vi "SteuerungWaermepumpe_DhruvTest.vi"() -> ()   [LabVIEW 2015]
uses:
  <vilib>/DAQmx/read.llb/DAQmx Read (Analog 1D Wfm NChan NSamp).vi
  <vilib>/DAQmx/write.llb/DAQmx Write (Analog 1D Wfm NChan 1Samp).vi
  <vilib>/MakerHub/LINX/Public/Peripherals/Digital/Digital Write N Chans.vi
  <vilib>/MakerHub/LINX/Private/Local IO/LinxDigitalWrite.vi
  <vilib>/MakerHub/LINX/Public/Utilities/Check Channel.vi
  <vilib>/MakerHub/LINX/Private/Utilties/Generate Error.vi
  <vilib>/DAQmx/miscellaneous.llb/DAQmx Fill In Error Info.vi
  <vilib>/Utility/file.llb/Read Delimited Spreadsheet (DBL).vi
  <vilib>/MakerHub/LINX/LMH-LINX.lvlib
panel:
  in  "stop":bool
  out "x = y?":bool
  out "concatenated string":string
  out "Number of Thermocouples":dbl
  out "Keithley Temperature Graph":waveform(dbl)[](graph)
  out "error out":errorcluster
  out "Array 2":dbl[](array[numeric])
  out "Abscheider":cluster{dbl, dbl, dbl}(slide) scale=0.0..1.3
  in  "Rampe":bool=TRUE
  in  "Rampe rpm/s":dbl=1.0 min=1.0 max=100.0 step=1.0
  out "Rampe IW":dbl
  in  "reinitialize HD":bool
  in  "reinitialize Pumpe":bool
  out "ist an!":string
  in  "zusätzlicher Druck":dbl
  in  "PI05 SW":dbl format="%.2f"
  out "p_liq_mittel":dbl
  out "p_liq":dbl
  out "Schleifendauer":dbl format="%.5f"
  out "Mittelwert 2":dbl
  in  "Mittelwert HD":bool
  in  "Mittelwert Pumpe":bool
  out "Mittelwert":dbl
  in  "Xi / p_liq berechnung an":bool
  out "xi_r":dbl
  in  "Regler Senke":bool
  in  "reinitialize Senke":bool
  in  "TI35 SW":dbl=43.0 format="%.2f"
  in  "Drehzahl Bestätigung":bool
  in  "Drehzahl SW":dbl=1000.0 min=500.0 max=3000.0 step=1.0 format="%#_4g"
  out "Check":dbl format="%#_13g"
  in  "Regler Hochdruck":bool
  in  "PID Regelung Pumpe":bool
  in  "SW TI39":dbl
  out "Array":bool[](array[boolean])
  in  "LEDs 2":bool[](array[boolean])
  in  "Regelung HK":bool
  in  "RV 30 zu":bool
  in  "RV 30 auf":bool
  out "FI_Oel":dbl
  in  "RV 33":dbl(slide) scale=-1.0..1.0
  in  "tag":string
  out "Pumpenwerte":dbl[](array[numeric]) format="%.2f"
  out "Speichert!":bool
  out "Historie":string
  in  "Kommentar":string
  out "refnum out":refnum<file>
  in  "Identität!":string(combo)
  in  "Zeit X in Minuten":dbl(slide)=5.0 min=0.0 max=15.0 scale=5.0..15.0
  out "TI 21a Warnungen":dbl
  out "Leistung":dynamicdata(graph)
  out "TI 37":dbl
  in  "Programm stoppen!":bool
  out "%":sgl(slide) scale=0.0..100.0
  out "kalt":bool
  out "warm":bool
  out "?":T1(array[cluster]) {"?" format="%#.4g"; "Konzentration_reich" format="%#.4g"}
  in  "Mit EES vergleichen":bool
  in  "FI13 SW in l/min":dbl=3.0 min=3.0 max=12.0 step=0.10000000149011612
  out "COP_Oel":dbl
  out "Q-Oel kW":dbl format="%_4g"
  in  "Dateiname!":string
  in  "Comment":bool
  in  "Speichern":bool caption="Aktivieren"
  out "ZU     Ventilstellung 33     AUF":dbl(slide) scale=0.0..100.0 scale format="%.2f"
  in  "Regelventil 34":dbl(slide) min=0.0 max=100.0 step=0.009999999776482582 scale=0.0..100.0
  in  "Matlab":bool
  in  "?":T2(tab)
  out "?":dynamicdata(graph)
  out "?":waveform(dbl)(graph)
  out "?":dynamicdata(graph)
  out "PI 12":dbl format="%.2f"
  out "PI 11":dbl format="%.2f"
  out "Dichte":dbl format="%.5g"
  in  "Reset":bool
  out "Betriebszeit":cluster{"second":i32, "minute":i32, "hour":i32}
  out "Temperatur Ölprüfstand":dbl
  out "FI 13 kg/min":dbl
  in  "Messung\nFrequenzwandler":bool
  out "Magnetventil":bool
  out "Fl.Pumpe an":bool
  out "Temperatur Öl":bool
  out "COP":dbl format="%#_13g"
  out "Verdichteraktivität":cluster{"second":i32, "minute":i32, "hour":i32}
  out "Q-Entgaser kW":dbl format="%_4g"
  out "Warnungen":bool[](array[boolean])
  out "Status Komponenten":bool[](array[boolean])
  in  "Pumpen-Auto-Abschalt":bool=TRUE
  out "Q-Resorber kW":dbl format="%_4g"
  out "Stellung Expansionsventil":waveform(dbl)(graph)
  out "FI 35 l/min":dbl format="%#_13g"
  out "FI 38 l/min":dbl format="%#_13g"
  out "FI Oel l/min":dbl format="%#.3g"
  out "LI in l":dbl format="%#_4g"
  out "TI 39":dbl format="%#_3g"
  out "TI 38":dbl format="%#_3g"
  out "TI 36":dbl format="%#_3g"
  out "TI 35":dbl format="%#_3g"
  out "TI 33":dbl format="%#_3g"
  out "TI 32":dbl format="%#_3g"
  out "TI 34":dbl format="%#_3g"
  out "TI 21a":dbl format="%#_3g"
  out "TI 21":dbl format="%#_3g"
  out "TI 20":dbl format="%#_3g"
  out "TI 14a":dbl format="%#_3g"
  out "TI 14":dbl format="%#_3g"
  out "TI 13":dbl format="%#_3g"
  out "TI 12":dbl format="%#_3g"
  out "TI 11":dbl format="%#_3g"
  out "TI 10":dbl format="%#_3g"
  out "TI 09":dbl format="%#_3g"
  out "TI 08":dbl format="%#_3g"
  out "TI 07":dbl format="%#_3g"
  out "TI 06a":dbl format="%#_3g"
  out "TI 06":dbl format="%#_3g"
  out "TI 05":dbl format="%#_3g"
  out "TI 04":dbl format="%#_3g"
  out "TI 22":dbl format="%#_3g"
  out "TI 02":dbl format="%#_3g"
  out "TI 01":dbl format="%#_3g"
  out "Konzentration":dbl format="%#_5g"
  in  "Pumpensteuerung":dbl min=0.0 max=10.0 step=0.009999999776482582 format="%.2g"
  out "PI 08":dbl format="%.2f"
  out "PI 05":dbl format="%#.2f"
  out "PI 02":dbl format="%.2f"
  out "PI 04":dbl format="%.2f"
  out "PDI 8-9":dbl format="%.2f"
  out "PI 14":dbl format="%.2f"
  out "PI 01":dbl format="%.2f"
  out "ZU    Ventilstellung Exp.V     AUF":dbl(slide) scale=0.0..100.0 scale format="%#.1f"
  in  "Exp.V":dbl(slide)=3.0 min=0.0 max=100.0 step=1.0 scale=0.0..100.0 scale format="%#.0f"
  out "ZU    Ventilstellung 14      AUF":dbl(slide) caption="Auf    Ventilstellung 14      Zu" scale=0.0..100.0 scale format="%#.2f"
  in  "Regelventil 36":dbl(slide) min=0.0 max=100.0 step=0.009999999776482582 scale=0.0..100.0 scale format="%#.0f"
  out "ZU  Ventilstellung 35  AUF":dbl(slide) scale=0.0..100.0 scale format="%.2f"
  in  "Regelventil 35":dbl(slide)=100.0 min=0.0 max=100.0 step=0.009999999776482582 scale=0.0..100.0 scale format="%#.3g"
  out "ZU     Ventilstellung 39     AUF":dbl(slide) scale=0.0..100.0 scale format="%.2f"
  in  "Regelventil 39":dbl(slide)=100.0 min=0.0 max=100.0 step=0.009999999776482582 scale=0.0..100.0
  out "FI 13 l/min":dbl format="%.2f"
  out "FI 07 l/min":dbl format="%.2f"
  out "LI in m":dbl format="%.2f"
  out "PDI 5-6":dbl format="%.4f"
  out "PI 07":dbl format="%.2f"
  out "Druckverhältnis":dbl
  out "Drehzahl":dbl
  out "Drehmoment":dbl
  out "Frequenz":dbl
  out "Leistung":dbl
  out "Durchfluss":waveform(dbl)[](graph)
  in  "Tab Control Temperaturen":T3(tab)
  out "Temperatur Reich":waveform(dbl)[](graph)
  out "Temperatur Arm":waveform(dbl)[](graph)
  out "Temperatur Öl":waveform(dbl)[](graph)
  out "Temperatur Senke/Quelle":waveform(dbl)[](graph)
  out "Druck":waveform(dbl)[](graph)
  out "Druckzustand":bool caption="Zu viel Druck !!!"
  # "Öltemperatur"
  # "Resorber"
  # "Entgaser"
  # "Druckverhältnis"
  # "ExpV"
  # "Verdichter an"
  # "iWÜ"
  # "Magnetventil"
  # "RV 39"
  # "RV 35"
  # "RV 33"
  # "RV 34"
  # "Pumpe an"
  # "Ölabscheider"
  # "2"
  # "1"
  # "RV 30"
  # "Verdichter"
  # "Pumpe"
  # "Leistung"
  # "kW"
  # "Speed"
  # "rpm"
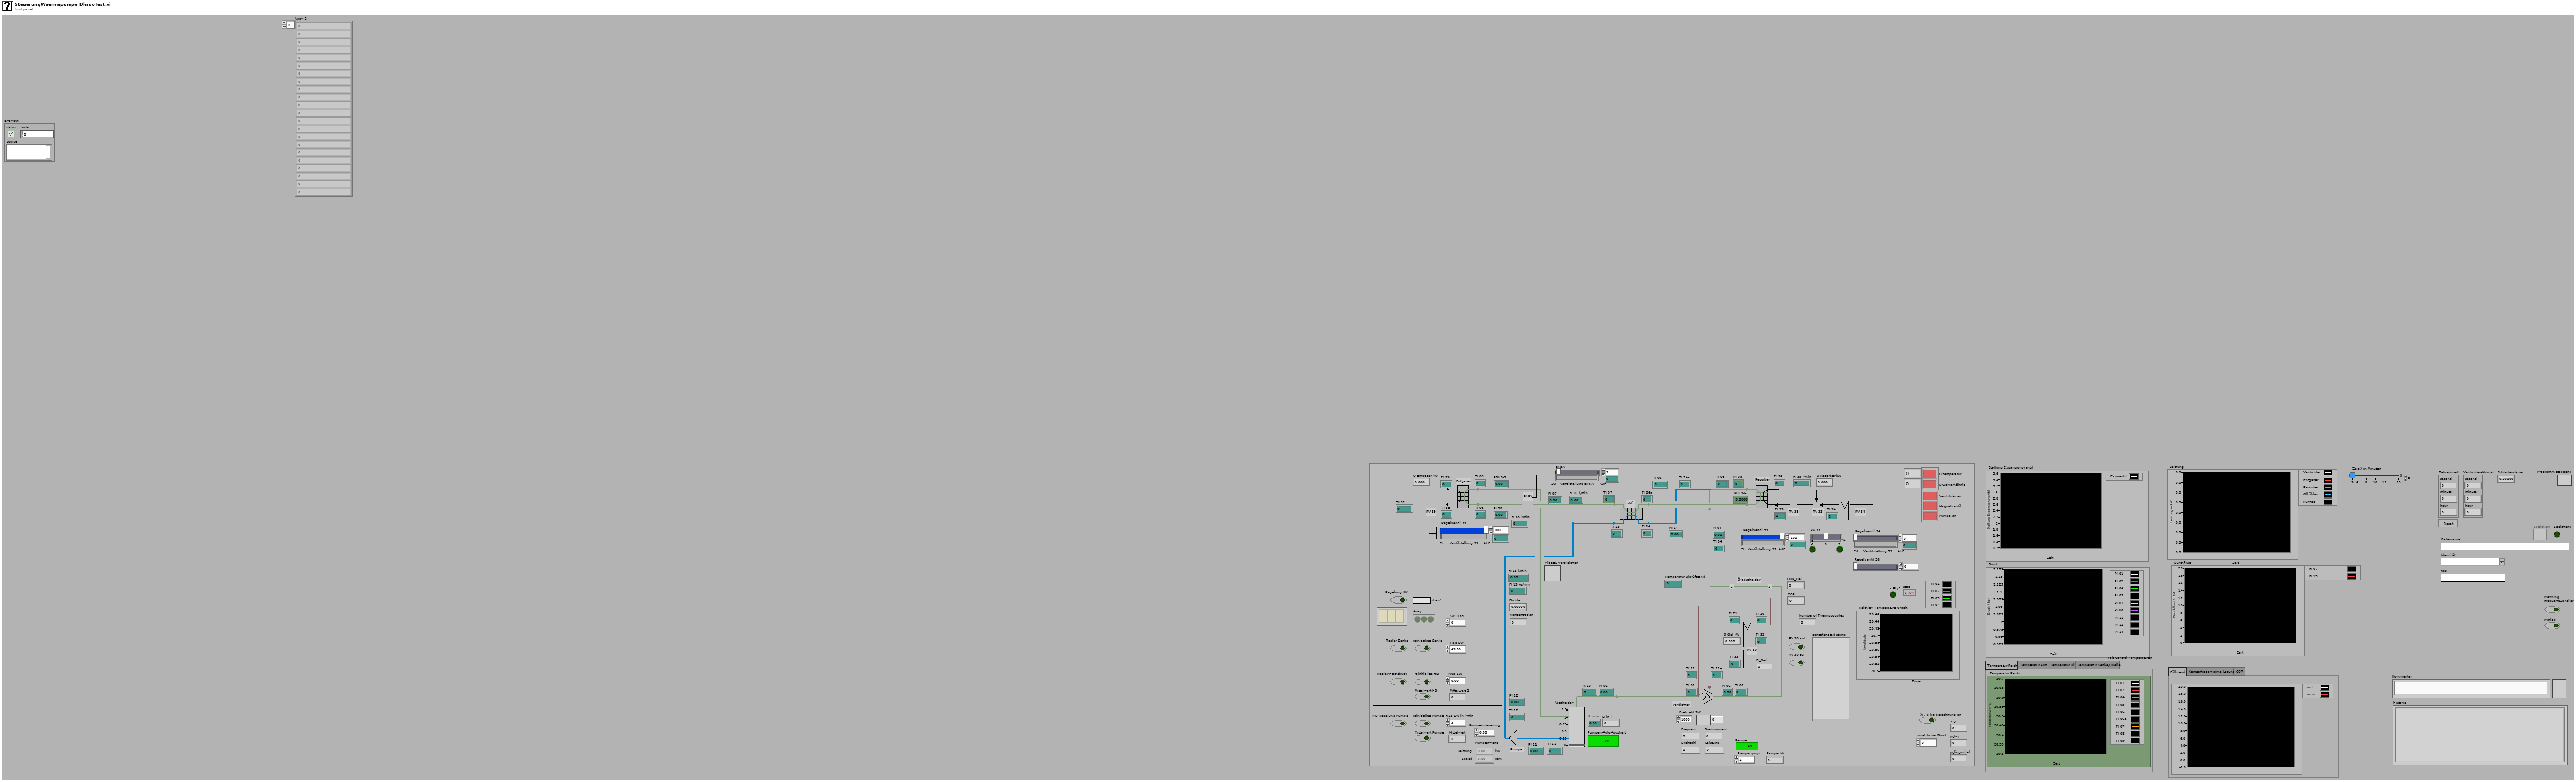
[diagram p1: front panel]
types:
  T1 = cluster{dbl, "Konzentration_reich":dbl, "String":string, bool}[]
  T2 = enum32{"Füllstand", "Konzentration arme Lösung", "COP"}
  T3 = enum32{"Temperatur Reich", "Temperatur Arm", "Temperatur Öl", "Temperatur Senke/Quelle"}
  T4 = enum8{"Enabled", "Disabled", "Disabled and Grayed Out"}
  T5 = typedef "LMH-LINX.lvlib/LINX Ref.ctl" = cluster{"IO":T6, "Interface":T7, "LINX Device Config":T8}
  T6 = typedef "LMH-LINX.lvlib/Platform.ctl" = enum16{"Remote", "Local"}
  T7 = typedef "LMH-LINX.lvlib/Interface.ctl" = enum16{"Serial", "TCP"}
  T8 = typedef "LMH-LINX.lvlib/Device.lvlib/LINX Device Config.ctl" = cluster{"Interface":T7, "COM Port":refnum<visa-resource-name>, "TCP Configuration":T9, "Device Family":u8, "Device ID":u8, "Device Name":string, "TCP Ref":refnum<k5>, "Channels":T10}
  T9 = typedef "LMH-LINX.lvlib/Device.lvlib/TCP Config.ctl" = cluster{"IP Address":string, "Port":u16}
  T10 = typedef "LMH-LINX.lvlib/Channels.ctl" = cluster{"DI":u8[], "DO":u8[], "AI":u8[], "AO":u8[], "PWM":u8[], "QE":u8[], "UART":u8[], "I2C 2":u8[], "SPI":u8[], "CAN":u8[], "Servo":u8[], "AI Ref (V)":dbl, "AI Resolution (Bits)":u8, "AO Ref (V)":dbl, "AO Resolution (Bits)":u8}
  T11 = enum16{"open", "replace", "create", "open or create", "replace or create", "replace or create with confirmation"}
  T12 = cluster{"Array[0]":dbl, "Array[1]":dbl, "Array[2]":dbl}
  T13 = cluster{"Array[0]":sgl, "Array[1]":sgl, "Array[2]":sgl}
  T14 = cluster{"Numeric":dbl, "Konzentration_reich":dbl, "String":string, bool}[]
  T15 = typedef "LVDateTimeRec.ctl" = cluster{"fractional second":dbl, "second":i32, "minute":i32, "hour":i32, "day of month":i32, "month":i32, "year":i32, "day of week":i32, "day of year":i32, "DST":i32}
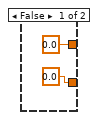
[diagram p8: hidden frame]
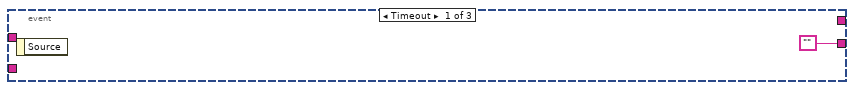
[diagram p10: hidden frame]
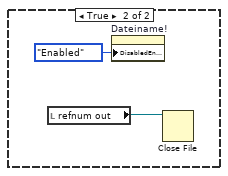
[diagram p11: hidden frame]
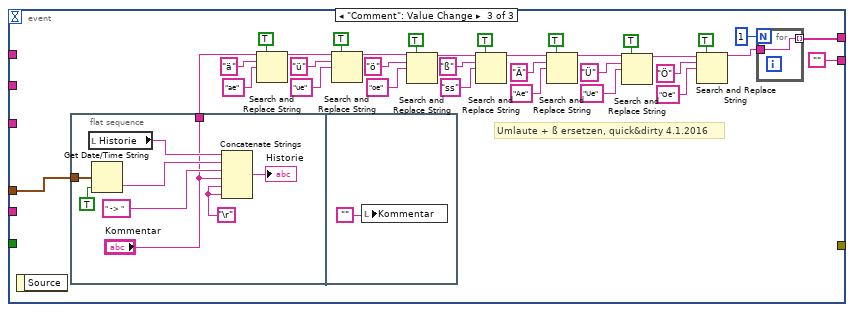
[diagram p12: hidden frame]
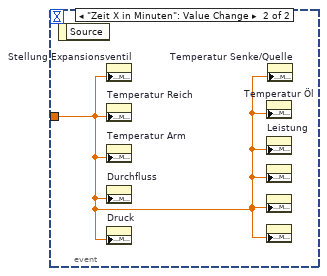
[diagram p13: hidden frame]
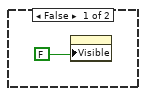
[diagram p14: hidden frame]
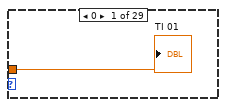
[diagram p17: hidden frame]
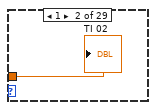
[diagram p18: hidden frame]
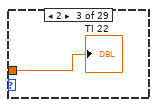
[diagram p19: hidden frame]
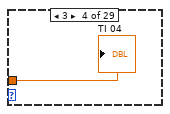
[diagram p20: hidden frame]
diagram:
  w26 = 10.0  # timeout (s)
  w25 = 1  # number of samples
  w38 = i32[] [8, 9, 10]  # Digital Output PIns
  w1 = FALSE ("Programm stoppen!")
  # "Final Thermocouple ID# (String)"
  # "First Thermocouple ID# (String)"
  # "Output_Task"
  # "Druck_Task"
  # "Temp_Task"
  # "Steuerung für Heizkerzen"
  # "Startbedingungen"
  n1 = call "Concat_Strings.vi"("Final Thermocouple ID# (String)"="103", "First Thermocouple ID# (String)"="102") -> ("Number of Thermocouples"=w4:dbl, "concatenated string"=w6:string)  [unwired: 8 in]
  "Number of Thermocouples" <- w4
  "concatenated string" <- w6
  n2 = Equal?(x="TRAC:CLE\n\n*RST\n\nTRAC:CLE:AUTO OFF\n\nSENS:FUNC 'TEMP',(@101:137)\n\nUNIT:TEMP C\n:TEMP:NPLC 1,(@101:137)\n\n:TEMP:TRAN FRTD,(@101)\n\n:TEMP:TRAN TC,(@101:137)\n:TEMP:TC:TYPE K,(@101:137)\n:TEMP:RJUN:RSEL INT,(@101:137)\n\nSAMP:COUN 37\nROUT:SCAN  (@101:137)\nINIT:CONT OFF\n\nTRIG:SOUR IMM\nTRIG:COUN 1\nTRIG:DEL:AUTO ON\n\nROUT:SCAN:TSO IMM\nROUT:SCAN:LSEL INT\n", y=w6) -> (x = y?=→"x = y?":bool)
  n3 = VISA Write(VISA resource name=refnum<visa-resource-name> "COM3", write buffer=w6) -> (VISA resource name out=w12:refnum<visa-resource-name>, error out=w13:errorcluster)  [unwired: 1 in, 1 out]
  n4 = flat-sequence {
    tunnel: w13 -> [w55]
    tunnel: [w55] -> w10
    tunnel: w12 -> [w53]
    tunnel: [w53] -> w11
    frame #0 {
      n5 = Wait (ms)(milliseconds to wait=u32 200 ("Zu wartende ms")) -> ()  [unwired: 1 out]
    }
  }
  n6 = Add(x=1.0, y=w4) -> (x+y=w2:dbl)
  n7 = while {
    tunnel: w11 -> [w67]
    tunnel: w10 -> [w66]
    tunnel: w2 -> [w64]
    stop <- "stop" stop-if-true
    n8 = flat-sequence {
      tunnel: [w94] -> w86
      tunnel: w66 -> [w91]
      tunnel: [w96] -> w85
      tunnel: w64 -> [w94]
      tunnel: w67 -> [w95]
      tunnel: [w90] -> w57
      tunnel: w86 -> [w99]
      tunnel: [w99] -> w84
      tunnel: [w98] -> w83
      tunnel: w85 -> [w98]
      tunnel: w57 -> [w97]
      tunnel: [w97] -> w56
      tunnel: w84 -> [w104]
      tunnel: [w104] -> w82
      tunnel: w83 -> [w106]
      tunnel: [w105] -> w81
      tunnel: [w103] -> w58
      tunnel: w56 -> [w102]
      tunnel: w82 -> [w110]
      tunnel: [w110] -> w80
      tunnel: w81 -> [w109]
      tunnel: [w109] -> w79
      tunnel: [w107] -> w59
      tunnel: w58 -> [w107]
      tunnel: w80 -> [w113]
      tunnel: [w113] -> w78
      tunnel: [w117] -> w77
      tunnel: [w116] -> w76
      tunnel: [w115] -> w75
      tunnel: w79 -> [w112]
      tunnel: w59 -> [w111]
      tunnel: w78 -> [w123]
      tunnel: [w122] -> w61
      tunnel: w77 -> [w121]
      tunnel: w76 -> [w120]
      tunnel: w75 -> [w124]
      tunnel: [w121] -> w69
      tunnel: [w120] -> w68
      frame #0 {
        n9 = Format Into String(format string="%.0f", w94) -> (resulting string=w89:string)  [unwired: 2 in, 1 out]
        n10 = Concatenate Strings("TRAC:CLE:AUTO ON\nTRAC:POIN ", w89, "\nTRAC:FEED SENS\nTRAC:FEED:CONT NEXT\nINIT\n" ("Daten")) -> (w87:string)
        n11 = VISA Write(VISA resource name=w95, write buffer=w87, error in (no error)=w91) -> (VISA resource name out=w96:refnum<visa-resource-name>, error out=w90:errorcluster)  [unwired: 1 out]
      }
      frame #1 {
        n12 = Wait (ms)(milliseconds to wait=u32 1600 ("ms Wartezeit")) -> ()  [unwired: 1 out]
      }
      frame #2 {
        n13 = VISA Write(VISA resource name=w106, write buffer="FORM:ELEM READ\nTRAC:DATA?\n", error in (no error)=w102) -> (VISA resource name out=w105:refnum<visa-resource-name>, error out=w103:errorcluster)  [unwired: 1 out]
      }
      frame #3 {
        n14 = Wait (ms)(milliseconds to wait=u32 200 ("ms Wartezeit")) -> ()  [unwired: 1 out]
      }
      frame #4 {
        n15 = property class="Instr"(reference=w112, error in=w111) -> (reference out=w118:refnum<visa-resource-name>, error out=w119:errorcluster, "Bytes at Port"=w114:u32)
        n16 = VISA Read(VISA resource name=w118, byte count=w114, error in (no error)=w119) -> (VISA resource name out=w117:refnum<visa-resource-name>, read buffer=w115:string, error out=w116:errorcluster)  [unwired: 1 out]
      }
      frame #5 {
        n17 = Initialize Array(0.0 ("Elementdaten"), w123) -> (w129:dbl[])
        n18 = Concatenate Strings(w124, "," ("Sub-Sring")) -> (w126:string)
        n19 = for {
          N: w123 -> [_]
          shift-right: [w139] -> w122
          shift-left: w129 -> [w130]
          shift-right: [w132] -> _
          shift-left: w126 -> [w138]
          shift-right: [w133] -> _
          shift-left: 0 -> [w134]
          n20 = Increment(x=w134) -> (x+1=w133:i32)
          n21 = Match Pattern(string=w138, regular expression="," ("gültiger Ausdruck")) -> (before substring=w135:string, after substring=w132:string)  [unwired: 1 in, 2 out]
          n22 = Fract/Exp String To Number(use system decimal point (T)=FALSE ("verwende System-Dezimalpunkt (T)"), string=w135) -> (number=w136:dbl)  [unwired: 2 in, 1 out]
          n23 = Replace Array Subset(array=w130, new element=w136, index=w134) -> (w139:dbl[])
        }
      }
    }
    n24 = VISA Close(VISA resource name=w69, error in (no error)=w68) -> (error out=→"error out":errorcluster)
    n25 = Get Date/Time In Seconds() -> (seconds since 1Jan1904=w62:timestamp)
    n26 = Spreadsheet String To Array(delimiter (Tab)=",", format string="%.3f", spreadsheet string="TI 01,TI 02,TI 03,TI 04,TI 05,TI 06,TI 07,TI 08,TI 09,TI 10,TI 11,TI 12,TI 13,TI 14,TI 15,TI 16,TI 17,TI 18,TI 19,TI 20,TI 21,TI 22,TI 23,TI 24,TI 25,TI 26,TI 27,TI 28,TI 29,TI 30,TI 31,TI 32,TI 33,TI 34,TI 35,TI 36,TI 37,TI 38,TI 39,TI 40", array type (2D Dbl)=string[] []) -> (array=w72:string[])
    n27 = for {
      tunnel: w72 -> [w145] mode=indexing
      tunnel: [w142] -> w65 mode=indexing
      tunnel: w62 -> [w141]
      tunnel: w61 -> [w140] mode=indexing
      n28 = Build Array(w140) -> (w144:dbl[])
      n29 = Bundle By Name("Y"=w144, "t0"=w141) -> (w143:waveform(dbl))  [unwired: 1 in]
      n30 = Set Waveform Attribute(5:w145, 6:"NI_ChannelName", 7:w143) -> (3:w142:waveform(dbl))  [unwired: 1 in, 2 out]
    }
    "Keithley Temperature Graph" <- w65
    "Array 2" <- w61
  }
  n31 = local write "Programm stoppen!"(w1) -> ()
  n32 = local write "Zeit X in Minuten"(5.0 ("Zeit X in Minuten")) -> ()
  n33 = local write "Historie"("") -> ()
  n34 = local write "Speichert!"(FALSE ("Speichert!")) -> ()
  n35 = local write "Speichern"(FALSE ("Speichern")) -> ()
  n36 = local write "ist an!"("") -> ()
  n37 = local write "Dateiname!"("") -> ()
  n38 = call <vilib>:"Initialize.vi"("Serial Port"=refnum<visa-resource-name> "COM4", "Error In"=errorcluster {"status"=FALSE, "code"=0, "source"=""}) -> ("Error Out"=w39:errorcluster, "Device Name"=w36:string, "LINX Resource"=w42:T5)  [unwired: 7 in]
  n39 = while {
    tunnel: w42 -> [w149]
    tunnel: [w159] -> w41
    tunnel: [w158] -> w40
    tunnel: w39 -> [w148]
    tunnel: w38 -> [w157]
    tunnel: w36 -> [w147]
    stop <- w156 stop-if-true
    n40 = local read "TI 39"() -> (w150:dbl)
    n41 = call "Filter6"("Signal"=w150) -> ("Filtered Signal"=w151:dynamicdata)  [unwired: 9 in, 1 out]
    n42 = call "Quellenregler.vi"("Regelung Quelle"="Regelung HK", "TI 38 IW °C"=w151, "LEDs"="LEDs 2", "TI 38 SW °C"="SW TI39") -> ("Kerzen von Regler"=w153:bool[])  [unwired: 3 in, 1 out]
    "Array" <- w153
    n43 = local read "Programm stoppen!"() -> (w156:bool)
    n44 = call-poly <vilib>:"Digital Write.vi"("Error In"=w148, "Values"=w153, "DO Channels"=w157, "LINX Resource"=w149) -> ("Error Out"=w158:errorcluster, "LINX Resource"=w159:T5)  [unwired: 6 in]
    "ist an!" <- w147
  }
  n45 = property on="Dateiname!" class="Str"("DisabledEnum"=T4."Enabled" ("Disabled")) -> ()  [unwired: 2 in, 2 out]
  n46 = local write "stop"(w1) -> ()
  n47 = call "DAQ_Pressure_Task.vi"() -> ("error out"=w30:errorcluster, "task out"=w31:refnum<k21>)  [unwired: 10 in]
  n48 = call "DAQ_Temp_Task.vi"() -> ("error out"=w32:errorcluster, "task out"=w33:refnum<k21>)  [unwired: 10 in]
  n49 = call <vilib>:"DAQmx Start Task.vi"("task/channels in"=w31, "error in"=w30) -> ("task out"=w24:refnum<k21>, "error out"=w27:errorcluster)  [unwired: 12 in]
  n50 = call <vilib>:"DAQmx Start Task.vi"("task/channels in"=w33, "error in"=w32) -> ("task out"=w28:refnum<k21>, "error out"=w29:errorcluster)  [unwired: 12 in]
  n51 = call <vilib>:"Close.vi"("Error In"=w40, "LINX Resource"=w41) -> ("Error Out"=w43:errorcluster)  [unwired: 9 in]
  n52 = call <vilib>:"Simple Error Handler.vi"("error in (no error)"=w43) -> ()  [unwired: 4 in, 5 out]
  n53 = call "DAQ_Output_Task.vi"() -> ("error out"=w18:errorcluster, "task out"=w19:refnum<k21>)  [unwired: 10 in]
  n54 = while {
    tunnel: [w194] -> w47
    tunnel: [w193] -> w16
    tunnel: w29 -> [w187]
    tunnel: w26 -> [w185]
    tunnel: w28 -> [w182]
    tunnel: w25 -> [w180]
    tunnel: w27 -> [w178]
    tunnel: w26 -> [w177]
    tunnel: w25 -> [w175]
    tunnel: w24 -> [w173]
    tunnel: [w169] -> w23
    tunnel: [w168] -> w22
    tunnel: [w166] -> w21
    tunnel: [w164] -> w20
    tunnel: w19 -> [w163]
    tunnel: w18 -> [w160]
    stop <- w192 stop-if-true
    n55 = flat-sequence {
      tunnel: [w205] -> w188
      tunnel: w187 -> [w204]
      tunnel: [w204] -> w186
      tunnel: w185 -> [w203]
      tunnel: [w203] -> w184
      tunnel: w182 -> [w202]
      tunnel: [w202] -> w183
      tunnel: [w201] -> w181
      tunnel: w180 -> [w201]
      tunnel: [w200] -> w179
      tunnel: w178 -> [w200]
      tunnel: w177 -> [w199]
      tunnel: [w199] -> w176
      tunnel: w175 -> [w198]
      tunnel: [w198] -> w174
      tunnel: w173 -> [w197]
      tunnel: [w197] -> w172
      tunnel: w163 -> [w196]
      tunnel: [w196] -> w162
      tunnel: [w195] -> w161
      tunnel: w160 -> [w195]
      tunnel: ["Programm stoppen!"] -> w192
      tunnel: [w424] -> w191
      tunnel: [w423] -> w190
      tunnel: [w227] -> w189
      tunnel: w188 -> [w227]
      tunnel: w186 -> [w265]
      tunnel: w184 -> [w264]
      tunnel: w183 -> [w263]
      tunnel: w181 -> [w262]
      tunnel: w179 -> [w261]
      tunnel: w176 -> [w260]
      tunnel: w174 -> [w259]
      tunnel: w172 -> [w258]
      tunnel: [w257] -> w171
      tunnel: [w256] -> w170
      tunnel: [w255] -> w167
      tunnel: [w254] -> w165
      tunnel: w162 -> [w252]
      tunnel: w161 -> [w251]
      tunnel: [w835] -> w193
      tunnel: [w836] -> w194
      tunnel: w191 -> [w836]
      tunnel: w190 -> [w835]
      tunnel: w189 -> [w833]
      tunnel: w171 -> [w828]
      tunnel: w170 -> [w829]
      tunnel: [w829] -> w169
      tunnel: [w828] -> w168
      tunnel: w167 -> [w827]
      tunnel: [w827] -> w166
      tunnel: w165 -> [w826]
      tunnel: [w826] -> w164
      frame #0 {
        n56 = Tick Count (ms)() -> (millisecond timer value=w205:u32)
      }
      frame #1 {
        w229 = 8.0  # Time Target
        w253 = TRUE  # auto start
        w443 = sgl 1.0
        w456 = 22
        w461 = 20
        w487 = -4
        w488 = 0
        # "RunningTime"
        # "TimeCountV"
        # "TimeCount"
        # "ENTE!"
        # "Sicherheiten für den Verdichter"
        # "Pumpenregelung PID"
        # "Skalierung der Graphen"
        # "Leistung Pumpe"
        # "Leistung"
        # "Durchfluss & Druck Anzeigen"
        # "Temperatur Anzeigen"
        # "Plots errechneter Größen"
        # "EES-Vergleich"
        # "Matlab-Skripte"
        # "Warnungen"
        # "Namensvergebung"
        # "Wärmestrom & COP"
        # "Notabschaltung Pumpe"
        # "Auslesen FU"
        # "Durchfluss & Druck Plot"
        # "Temperatur Plot"
        # "Aufzeichnung Protokoll"
        # "Variable Stellungen"
        n57 = call-poly <vilib>:"DAQmx Read.vi"("task/channels in"=w258, "number of samples per channel"=w259, "timeout"=w260, "error in"=w261) -> ("task out"=w257:refnum<k21>, "data"=w267:waveform(dbl)[], "error out"=w254:errorcluster)  [unwired: 9 in]
        n58 = call-poly <vilib>:"DAQmx Read.vi"("task/channels in"=w263, "number of samples per channel"=w262, "timeout"=w264, "error in"=w265) -> ("task out"=w256:refnum<k21>, "data"=w266:waveform(dbl)[], "error out"=w255:errorcluster)  [unwired: 9 in]
        n59 = call "Convert from Dynamic Data2"("Dynamic Data Type"=w267) -> ("Array"=w272:dbl[])  [unwired: 3 in]
        n60 = for {
          tunnel: w272 -> [w774] mode=indexing
          tunnel: [w773] -> w277 mode=indexing
          i -> [w775]
          n61 = case shown="19" w775 {
            tunnel: w774 -> [w776 w777 w778 w779 w780 w781 w782 w783 w784 w785 w786 w795 w807 w810 w811 w812 w813 w814 w817 w821 w822 w823 w824 w825 _]
            tunnel: [_ _ _ _ _ _ _ _ _ _ _ w787 _ _ _ _ _ _ w815 w819 _ _ _ _ _] -> w773
            frame 0 {
              "PI 01" <- w776
            }
            frame 1 {
              "PI 02" <- w777
            }
            frame 2 {
              "PI 04" <- w778
            }
            frame 3 {
              "PI 05" <- w779
            }
            frame 4 {
              "PI 07" <- w780
            }
            frame 5 {
              "PI 08" <- w781
            }
            frame 6 {
              "PI 11" <- w782
            }
            frame 7 {
              "PI 12" <- w783
            }
            frame 8 {
              "PI 14" <- w784
            }
            frame 9 {
              "PDI 5-6" <- w785
            }
            frame 10 {
              "PDI 8-9" <- w786
            }
            frame 11 {
              n62 = call "Filter3"("Signal"=w795) -> ("Filtered Signal"=w793:dynamicdata)  [unwired: 9 in, 1 out]
              n63 = Greater?(x=w795, y=0.3) -> (0:w790:bool)
              n64 = case shown="False" w790 {
                tunnel: w795 -> [_ w806]
                tunnel: [0.0 w806] -> w798
                frame False {
                }
                frame True {
                }
              }
              n65 = call "Convert from Dynamic Data6"("Dynamic Data Type"=w793) -> ("Scalar"=w792:dbl)  [unwired: 3 in]
              n66 = Multiply(x=w792, y=10.0) -> (x*y=w794:dbl)
              n67 = Greater?(x=w795, y=0.4) -> (0:w791:bool)
              n68 = formula code="float64 y; float64 Vu; /*Vu: Volumen schmaler Zylinder+Fuellstandsmesser*/\nVu=10;  /* 10 Liter */\n\nif (x<=10.25) \ny=(x-1)*pi*(0.536**2+0.32**2);\nelse\ny=Vu+(x-10.25)*pi*(1.584**2+0.32**2);"("x"=w794) -> ("y"=w787:dbl)
              "LI in l" <- w787
              n69 = case shown="False" w791 {
                tunnel: w795 -> [_ w804]
                tunnel: [0.0 w804] -> w797
                frame False {
                }
                frame True {
                }
              }
              n70 = Merge Signals(w795, w798, w797) -> (w799:dynamicdata)
              n71 = call "Convert from Dynamic Data3"("Dynamic Data Type"=w799) -> ("Array"=w802:dbl[])  [unwired: 3 in]
              n72 = Array To Cluster(array=w802) -> (cluster=w789:T12)
              n73 = To Single Precision Float(number=w789) -> (single precision float=→"Abscheider":T13)
              "LI in m" <- w795
            }
            frame 12 {
              "FI 07 l/min" <- w807
            }
            frame 13 {
              n74 = local read "Dichte"() -> (w809:dbl)
              n75 = Multiply(x=w810, y=w809) -> (x*y=→"FI 13 kg/min":dbl)
              "FI 13 l/min" <- w810
            }
            frame 14 {
              "ZU     Ventilstellung 39     AUF" <- w811
              "ZU     Ventilstellung 33     AUF" <- w811
            }
            frame 15 {
              "ZU  Ventilstellung 35  AUF" <- w812
            }
            frame 16 {
              # "RV14 ist entfernt"
              "ZU    Ventilstellung 14      AUF" <- w813
            }
            frame 17 {
              "ZU    Ventilstellung Exp.V     AUF" <- w814
            }
            frame 18 {
              n76 = call "Filter"("Signal"=w817) -> ("Filtered Signal"=w816:dynamicdata)  [unwired: 9 in, 1 out]
              n77 = call "Convert from Dynamic Data4"("Dynamic Data Type"=w816) -> ("Scalar"=w818:dbl)  [unwired: 3 in]
              n78 = formula code="float64 D;\nD=9.375*StromDichte+0.7125;\nD=floor(D*100000)/100000;"("StromDichte"=w818) -> ("D"=w815:dbl)
              "Dichte" <- w815
            }
            frame 19 {
              n79 = call "Filter2"("Signal"=w821) -> ("Filtered Signal"=w820:dynamicdata)  [unwired: 9 in, 1 out]
              n80 = To Double Precision Float(number=w820) -> (double precision float=w819:dbl)
              "Konzentration" <- w819
            }
            frame 20 {
              "FI Oel l/min" <- w822
            }
            frame 21 {
              "FI 38 l/min" <- w823
            }
            frame 22 {
              "FI 35 l/min" <- w824
            }
            frame 23 {
              "FI_Oel" <- w825
            }
            frame 24, Default {
            }
          }
        }
        n81 = call "Von dynamischen Daten konvertieren2"("Dynamic Data Type"=w266) -> ("Array"=w212:dbl[])  [unwired: 3 in]
        n82 = for {
          tunnel: i32[] [0, 1, 3, 4, 5, 6, 7, 8, 9] -> [w588] mode=indexing
          tunnel: w266 -> [w587]
          tunnel: [w586] -> w361 mode=indexing
          n83 = Index Array(array=w587, index=w588) -> (element=w586:waveform(dbl))
        }
        "Temperatur Reich" <- w361
        n84 = for {
          tunnel: i32[] [10, 11, 12, 13, 14, 15] -> [w585] mode=indexing
          tunnel: w266 -> [w584]
          tunnel: [w583] -> w362 mode=indexing
          n85 = Index Array(array=w584, index=w585) -> (element=w583:waveform(dbl))
        }
        "Temperatur Arm" <- w362
        n86 = for {
          tunnel: i32[] [16, 17, 18, 2] -> [w582] mode=indexing
          tunnel: w266 -> [w581]
          tunnel: [w580] -> w363 mode=indexing
          n87 = Index Array(array=w581, index=w582) -> (element=w580:waveform(dbl))
        }
        "Temperatur Öl" <- w363
        n88 = Index Array(array=w267, index=17) -> (element=→"Stellung Expansionsventil":waveform(dbl))
        n89 = for {
          tunnel: i32[] [19, 20, 21, 22, 23, 24, 25] -> [w579] mode=indexing
          tunnel: w266 -> [w578]
          tunnel: [w577] -> w364 mode=indexing
          n90 = Index Array(array=w578, index=w579) -> (element=w577:waveform(dbl))
        }
        "Temperatur Senke/Quelle" <- w364
        n91 = for {
          tunnel: [w573] -> w359 mode=indexing
          tunnel: w267 -> [w572]
          tunnel: i32[] [0, 1, 2, 3, 4, 5, 6, 7, 8] -> [w571] mode=indexing
          n92 = Index Array(array=w572, index=w571) -> (element=w573:waveform(dbl))
        }
        "Druck" <- w359
        n93 = for {
          tunnel: [w576] -> w360 mode=indexing
          tunnel: w267 -> [w575]
          tunnel: i32[] [12, 13] -> [w574] mode=indexing
          n94 = Index Array(array=w575, index=w574) -> (element=w576:waveform(dbl))
        }
        "Durchfluss" <- w360
        n95 = Get Date/Time In Seconds() -> (seconds since 1Jan1904=w226:timestamp)
        n96 = for {
          tunnel: w212 -> [w743] mode=indexing
          i -> [w744]
          n97 = case shown="17" w744 {
            tunnel: w743 -> [w745 w746 w747 w748 w749 w750 w751 w752 w753 w754 w755 w756 w757 w758 w759 w760 w761 w762 w763 w764 w765 w766 w767 w768 w769 w770 w771 w772 _]
            frame 0 {
              "TI 01" <- w745
            }
            frame 1 {
              "TI 02" <- w746
            }
            frame 2 {
              "TI 22" <- w747
            }
            frame 3 {
              "TI 04" <- w748
            }
            frame 4 {
              "TI 05" <- w749
            }
            frame 5 {
              "TI 06" <- w750
            }
            frame 6 {
              "TI 06a" <- w751
            }
            frame 7 {
              "TI 07" <- w752
            }
            frame 8 {
              "TI 08" <- w753
            }
            frame 9 {
              "TI 09" <- w754
            }
            frame 10 {
              "TI 10" <- w755
            }
            frame 11 {
              "TI 11" <- w756
            }
            frame 12 {
              "TI 12" <- w757
            }
            frame 13 {
              "TI 13" <- w758
            }
            frame 14 {
              "TI 14" <- w759
            }
            frame 15 {
              "TI 14a" <- w760
            }
            frame 16 {
              "TI 20" <- w761
            }
            frame 17 {
              "TI 21" <- w762
            }
            frame 18 {
              "TI 21a" <- w763
              "TI 21a Warnungen" <- w763
            }
            frame 19 {
              # "Check T_Heater"
              "TI 34" <- w764
            }
            frame 20 {
              "TI 32" <- w765
            }
            frame 21 {
              "TI 33" <- w766
            }
            frame 22 {
              "TI 35" <- w767
            }
            frame 23 {
              "TI 36" <- w768
            }
            frame 24 {
              "TI 38" <- w769
            }
            frame 25 {
              "TI 39" <- w770
            }
            frame 26 {
              "Temperatur Ölprüfstand" <- w771
            }
            frame 27 {
              "TI 37" <- w772
            }
            frame 28, Default {
            }
          }
        }
        n98 = To Double Precision Float(number=w226) -> (double precision float=w214:dbl)
        n99 = event shown="[0] Timeout" {
          selector: _ -> [_]
          dyn-events: _ -> [_]
          timeout: 2 -> [_]
          event Timeout {
            n100 = event-data() -> ()  [unwired: 1 in, 1 out]
          }
        }
        n101 = Index Array(array=w272, index #1=22 ("index"), index #2=23 ("index"), index #3=21 ("index")) -> (element #1=w394:dbl, element #2=w370:dbl, element #3=w393:dbl)
        n102 = Index Array(array=w212, index #1=22 ("index"), index #2=23 ("index"), index #3=21 ("index"), index #4=20 ("index"), index #5=25 ("index"), index #6=24 ("index")) -> (element #1=w392:dbl, element #2=w391:dbl, element #3=w390:dbl, element #4=w389:dbl, element #5=w388:dbl, element #6=w387:dbl)
        n103 = call "fu_gesamt.vi"("Boolean"="Messung\nFrequenzwandler") -> ("Frequenz"=w382:dbl, "Drehmoment"=w383:dbl, "Leistung"=w238:dbl, "Drehzahl"=w384:dbl, "Scaled"=w240:dbl[])  [unwired: 6 in]
        "Leistung" <- w238
        "Frequenz" <- w382
        "Drehmoment" <- w383
        "Drehzahl" <- w384
        "Pumpenwerte" <- w240
        n104 = call "Wärmestromrechner.vi"("Taus"=w391, "Tein"=w392, "Massenstrom"=w394) -> ("Wärmestrom Q"=w291:dbl)  [unwired: 2 in]
        "Q-Resorber kW" <- w291
        n105 = call "Wärmestromrechner.vi"("Taus"=w389, "Tein"=w390, "Massenstrom"=w370) -> ("Wärmestrom Q"=w278:dbl)  [unwired: 2 in]
        "Q-Oel kW" <- w278
        n106 = call "Wärmestromrechner.vi"("Taus"=w387, "Tein"=w388, "Massenstrom"=w393) -> ("Wärmestrom Q"=w290:dbl)  [unwired: 2 in]
        "Q-Entgaser kW" <- w290
        n107 = Index Array(array=w240, index=0) -> (element=w292:dbl)
        n108 = call "Set_timestamp.vi"("Eingang 5"=w292, "Eingang 4"=w278, "Eingang 3"=w291, "Eingang 2"=w290, "Eingang"=w238) -> ("Ausgang 4"=w288:waveform(dbl), "Ausgang 3"=w287:waveform(dbl), "Ausgang 2"=w286:waveform(dbl), "Ausgang"=w285:waveform(dbl), "Ausgang 5"=w289:waveform(dbl))  [unwired: 2 in]
        n109 = Merge Signals(w285, w286, w287, w288, w289) -> (→"Leistung":dynamicdata)
        n110 = formula code="float64 COP; float64 COP_Oel;\n\nCOP=Q/(Pp+Pv);\nCOP_Oel=(Q_Oel+Q)/(Pp+Pv);"("Pv"=w238, "Q"=w291, "Pp"=w292, "Q_Oel"=w278) -> ("COP"=w300:dbl, "COP_Oel"=w299:dbl)
        "COP" <- w300
        "COP_Oel" <- w299
        n111 = local read "Konzentration"() -> (w304:dbl)
        n112 = Empty Array?(array=w240) -> (empty?=w242:bool)
        n113 = local read "LI in m"() -> (w302:dbl)
        n114 = local read "LI in l"() -> (w301:dbl)
        n115 = Select(t=dbl[] [0.0, 0.0], s=w242, f=w240) -> (s? t:f=w239:dbl[])
        n116 = call "Set_timestamp.vi"("Eingang 5"=w304, "Eingang 4"=w302, "Eingang 3"=w301, "Eingang 2"=w300, "Eingang"=w299) -> ("Ausgang 4"=w297:waveform(dbl), "Ausgang 3"=w296:waveform(dbl), "Ausgang 2"=w294:waveform(dbl), "Ausgang"=w293:waveform(dbl), "Ausgang 5"=→"?":waveform(dbl))  [unwired: 2 in]
        n117 = Index Array(array=w277, index #1=18 ("index"), index #2=19 ("index"), index #3=11 ("index")) -> (element #1=w279:dbl, element #2=w276:dbl, element #3=w280:dbl)
        n118 = Merge Signals(w293, w294) -> (→"?":dynamicdata)
        n119 = Merge Signals(w296, w297) -> (→"?":dynamicdata)
        n120 = Build Array (concatenate)(w238, w384, w383, w382, w291, w290, w300, w279, w276, w280, w278, w239) -> (w211:dbl[])
        n121 = disable-structure shown="Disabled" {
          disable-tunnel: [w533 _] -> w484
          disable-tunnel: [w532 _] -> w473
          disable-tunnel: [w531 _] -> w462
          disable-tunnel: [w530 _] -> w386
          disable-tunnel: [w529 _] -> w381
          disable-tunnel: w370 -> [w528 _]
          disable-tunnel: w238 -> [w527 _]
          disable-tunnel: w272 -> [w526 _]
          disable-tunnel: w212 -> [w525 _]
          frame Disabled {
            n122 = call "Matlab-Calc.vi"("Temp-Array"=w525, "Matlab?"="Matlab", "Leistung"=w527, "Druck-Array"=w526, "FI Öl"=w528) -> ("m_reich [g/s]"=w532:dbl, "Konzentration_reich"=w529:dbl, "m_arm [g/s]"=w533:dbl, "Dampfmassenstrom [g/s]"=w530:dbl, "Dampfmassenanteil"=w531:dbl)  [unwired: 3 in, 7 out]
          }
          frame Enabled {
          }
        }
        n123 = Index Array(array=w272, index #1=0 ("index"), index #2=1 ("index"), index #3=2 ("index"), index #4=21 ("index"), index #5=22 ("index")) -> (element #1=w467:dbl, element #2=w468:dbl, element #3=w469:dbl, element #4=w466:dbl, element #5=w464:dbl)
        n124 = call "Temperaturen"("Signals"=w266) -> ("Signal Out"=w474:dynamicdata)  [unwired: 9 in, 1 out]
        n125 = call "Von dynamischen Daten konvertieren3"("Dynamic Data Type"=w474) -> ("Array"=w475:dbl[])  [unwired: 3 in]
        n126 = Build Array (concatenate)(w475, w299, w466, w484, w473, 1.0 ("element"), w386, w464, w469, w468, w467, 1.0 ("element"), 1.0 ("element"), 1.0 ("element"), w290, 1.0 ("element"), w291, w462, 1.0 ("element"), w276, w381) -> (w476:dbl[])
        n127 = Multiply(x=600, y="Zeit X in Minuten") -> (x*y=w435:dbl)
        n128 = event shown="[0] Timeout" {
          selector: _ -> [_ _]
          dyn-events: _ -> [_ _]
          timeout: 5 -> [_ _]
          tunnel: w435 -> [_ w717]
          event Timeout {
            n129 = event-data() -> ()  [unwired: 1 in, 1 out]
          }
          event "Zeit X in Minuten": Value Change {
            n130 = event-data() -> ()  [unwired: 1 in, 1 out]
            n131 = property on="Stellung Expansionsventil" class="WFChart (strict)"("XScale.Maximum"=w717) -> ()  [unwired: 2 in, 2 out]
            n132 = property on="Temperatur Reich" class="WFChart (strict)"("XScale.Maximum"=w717) -> ()  [unwired: 2 in, 2 out]
            n133 = property on="Temperatur Arm" class="WFChart (strict)"("XScale.Maximum"=w717) -> ()  [unwired: 2 in, 2 out]
            n134 = property on="Durchfluss" class="WFChart (strict)"("XScale.Maximum"=w717) -> ()  [unwired: 2 in, 2 out]
            n135 = property on="Druck" class="WFChart (strict)"("XScale.Maximum"=w717) -> ()  [unwired: 2 in, 2 out]
            n136 = property on="Temperatur Öl" class="WFChart (strict)"("XScale.Maximum"=w717) -> ()  [unwired: 2 in, 2 out]
            n137 = property on="Leistung" class="WFChart (strict)"("XScale.Maximum"=w717) -> ()  [unwired: 2 in, 2 out]
            n138 = property class="WFChart (strict)"("XScale.Maximum"=w717) -> ()  [unwired: 2 in, 2 out]
            n139 = property class="WFChart (strict)"("XScale.Maximum"=w717) -> ()  [unwired: 2 in, 2 out]
            n140 = property class="WFChart (strict)"("XScale.Maximum"=w717) -> ()  [unwired: 2 in, 2 out]
            n141 = property on="Temperatur Senke/Quelle" class="WFChart (strict)"("XScale.Maximum"=w717) -> ()  [unwired: 2 in, 2 out]
          }
        }
        n142 = case shown="True" "Mit EES vergleichen" {
          tunnel: w476 -> [_ w719]
          frame False {
            n143 = property class="Arr (strict)"("Visible"=FALSE) -> ()  [unwired: 2 in, 2 out]
          }
          frame True {
            # "K->C°"
            # "Toleranz"
            n144 = call-poly <vilib>:"Read Delimited Spreadsheet.vi"("file path (dialog if empty)"=path "Z:/HT-Waermepumpe/Projekte/SubVi_EES_vergleich/test.txt", "format (%.3f)"="%,;%.3f") -> ("first row"=w726:dbl[])  [unwired: 8 in, 5 out]
            n145 = Delete From Array(array=w726, length=20) -> (deleted portion=w722:dbl[], array with subset deleted=w724:dbl[])  [unwired: 1 in]
            n146 = expression code="x-273.15"(w724) -> (w723:dbl[])
            n147 = Insert Into Array(array=string[] ["T 01", "T 02", "T 04", "T 05", "T 06", "T 07", "T 08", "T 09", "T 10", "T 11", "T 12", "T 13", "T 14", "T 35", "T 36", "T 38", "T 39"] ("Array"), new element=string[] ["COP_Öl", "m_dot_ENT_W", "m_dot_LIQ", "m_dot_MIX", "m_dot_oil", "m_dot_VAP", "m_dot_RES_W", "p_HD", "P_KOMP", "p_ND", "P_PUMP_th", "P_KOMP_th", "Q_dot_ENT", "Q_dot_ENT_W", "Q_dot_oil", "Q_dot_RES_W", "q_geg", "Q_dot_RES", "xi_LIQ", "xi_MIX"] ("Array")) -> (w733:string[])  [unwired: 1 in]
            n148 = property class="Arr (strict)"("Visible"=TRUE) -> ()  [unwired: 2 in, 2 out]
            n149 = Insert Into Array(array=w723, new element=w722) -> (w720:dbl[])  [unwired: 1 in]
            n150 = expression code="x*0.05"(w720) -> (w721:dbl[])
            n151 = Add(x=w720, y=w721) -> (x+y=w729:dbl[])
            n152 = Subtract(x=w720, y=w721) -> (x-y=w728:dbl[])
            n153 = Greater Or Equal?(x=w729, y=w719) -> (x >= y?=w730:bool[])
            n154 = Less Or Equal?(x=w728, y=w719) -> (x <= y?=w731:bool[])
            n155 = And(x=w730, y=w731) -> (x .and. y?=w727:bool[])
            n156 = Build Cluster Array(w720, w719, w733, w727) -> (→"?":T14)
          }
        }
        n157 = Index Array(array=w272, index #1=2 ("index"), index #2=3 ("index"), index #3=4, index #4=5, index #5=11 ("index")) -> (element #1=w340:dbl, element #2=w339:dbl, element #3=w338:dbl, element #4=w344:dbl, element #5=w320:dbl)
        n158 = Build Array(w340, w339, w338) -> (w337:dbl[])
        n159 = Index Array(array=w212, index #1=19, index #2=w461, index #3=w456, index #4=23) -> (element #1=w453:dbl, element #2=w452:dbl, element #3=w451:dbl, element #4=w450:dbl)
        n160 = Index Array(array=w272, index #1=w461, index #2=w456) -> (element #1=w459:dbl, element #2=w458:dbl)
        n161 = Array Max & Min(array=w337) -> (min value=w233:dbl)  [unwired: 3 out]
        n162 = call "Filter5"("Signal"=w458) -> ("Filtered Signal"=w454:dynamicdata)  [unwired: 9 in, 1 out]
        n163 = call "Filter4"("Signal"=w459) -> ("Filtered Signal"=w455:dynamicdata)  [unwired: 9 in, 1 out]
        n164 = Less?(x=w233, y=20.5 ("x")) -> (x < y?=w231:bool)
        n165 = Greater Or Equal?(x=w233, y=18.5 ("x")) -> (x >= y?=w232:bool)
        "Druckzustand" <- w232
        n166 = call "Convert from Dynamic Data11"("Dynamic Data Type"=w455) -> ("Scalar"=w449:dbl)  [unwired: 3 in]
        n167 = call "Convert from Dynamic Data12"("Dynamic Data Type"=w454) -> ("Scalar"=w448:dbl)  [unwired: 3 in]
        n168 = formula code="float32 TIM1; float32 P; float32 H; float32 K;\nH=0; K=0;\nTIM1=((TI36*FI35)+(TI32*FIOel))/(FI35+FIOel);\nif((TI36-TI35) > 2) {\nif((TIM1-TI35) < (0.2)) {\nH=1;}\nelse {\nH=0;}\nif((TI35-TI30) < (0.2)) {\nK=1;}\nelse {\nK=0; }\nP=100/(TIM1-TI30)*(TI35-TI30);\n}"("TI30"=w453, "TI32"=w452, "TI35"=w451, "TI36"=w450, "FIOel"=w449, "FI35"=w448) -> ("H"=w447:sgl, "K"=w444:sgl, "P"=→"%":sgl)  [unwired: 1 out]
        n169 = feedback #1() -> (w223:dbl)  [unwired: 1 in]
        n170 = Select(t=w214, s=w231, f=w223) -> (s? t:f=w224:dbl)
        n171 = feedback-in #1(w224) -> ()
        n172 = case shown="True" "Pumpen-Auto-Abschalt" {
          tunnel: w320 -> [_ w740]
          frame False {
          }
          frame True {
            n173 = Less?(x=w740, y=0.3) -> (x < y?=w739:bool)
            n174 = case shown="True" w739 {
              frame False {
              }
              frame True {
                n175 = local write "Pumpensteuerung"(0.0) -> ()
              }
            }
          }
        }
        n176 = Subtract(x=w214, y=w224) -> (x-y=w230:dbl)
        n177 = Greater Or Equal?(x=w344, y=9.9 ("x")) -> (x >= y?=w348:bool)
        n178 = Greater Or Equal?(x=w230, y=w229) -> (x >= y?=w228:bool)
        n179 = Or(x=w228, y=w348) -> (x .or. y?=w330:bool)
        n180 = Or(x="Drehzahl Bestätigung", y=w330) -> (x .or. y?=w332:bool)
        n181 = case shown="True" w232 {
          frame False {
          }
          frame True {
            n182 = call <vilib>:"Play Sound File.vi"("path"=path "C:/Users/Hybrid/Desktop/ente_1.wav", "device ID"=u32 0) -> ()  [unwired: 8 in, 2 out]
          }
        }
        n183 = Equal?(x=w447, y=w443) -> (x = y?=→"warm":bool)
        n184 = Equal?(x=w444, y=w443) -> (x = y?=→"kalt":bool)
        n185 = feedback #2() -> (w331:dbl)  [unwired: 1 in]
        "Check" <- w331
        n186 = case shown="True" w330 {
          tunnel: w331 -> [w564 w568]
          tunnel: [w564 w569] -> w237
          frame False {
          }
          frame True {
            n187 = local write "Drehzahl SW"(1000.0) -> ()
            n188 = Multiply(x=w568, y=0.0) -> (x*y=w569:dbl)
            n189 = local write "Regler Hochdruck"(FALSE ("Regler Hochdruck")) -> ()
            n190 = local write "Exp.V"(60.0 ("Exp.V")) -> ()
          }
        }
        n191 = Select(t=0.0, s=w330, f="Drehzahl SW") -> (s? t:f=w334:dbl)
        n192 = feedback-in #2(w334, w332) -> ()
        n193 = local read "Konzentration"() -> (w210:dbl)
        n194 = case shown="True" "Rampe" {
          tunnel: [w520 w521] -> w236
          tunnel: w237 -> [w520 w523]
          frame False {
          }
          frame True {
            n195 = local read "Drehzahl"() -> (w522:dbl)
            n196 = formula code="if (ns > 100) {\nns=100;}\nif (ns < 1) {\nns=1;}\nif ((nSW>nSWR) &&  (nIW>=1000)) {\nnSWR=nSWR+ns;}\nelse {\nnSWR=nSW;}"("nSW"=w523, "ns"="Rampe rpm/s", "nIW"=w522) -> ("nSWR"=w521:dbl)
            "Rampe IW" <- w521
          }
        }
        n197 = case shown="True" "Xi / p_liq berechnung an" {
          tunnel: w212 -> [_ w563]
          tunnel: w272 -> [_ w556]
          tunnel: [0.0 w549] -> w322
          tunnel: [0.0 w546] -> w312
          tunnel: w211 -> [_ w544]
          tunnel: w210 -> [_ w543]
          frame False {
          }
          frame True {
            n198 = Index Array(array=w544, index=8) -> ()  [unwired: 1 out]
            n199 = Index Array(array=w556, index #1=4 ("index"), index #2=8 ("index")) -> (element #1=w551:dbl, element #2=w550:dbl)
            n200 = Index Array(array=w563, index #1=7 ("index"), index #2=6 ("index"), index #3=13 ("index"), index #4=14 ("index"), index #5=5 ("index")) -> (element #1=w555:dbl, element #2=w554:dbl, element #3=w553:dbl, element #4=w552:dbl, element #5=w547:dbl)
            n201 = script code="xi_a = xi_a/100;\ntry\nF = @(xi_r) ((refpropm('H','T',T6a+273.15,'P',p7*100,'ammonia','water',[xi_r 1-xi_r])*0.001-refpropm('H','T',T7+273.15,'P',p7*100,'ammonia','water',[xi_r 1-xi_r])*0.001)/(refpropm('H','T',T14+273.15,'P',p14*100,'ammonia','water',[xi_a 1-xi_a])*0.001-refpropm('H','T',T13+273.15,'P',p14*100,'ammonia','water',[xi_a 1-xi_a])*0.001)*(xi_a-1)+1-xi_r);\nxi_r0=xi_a;\n[xi_r, fval] = fzero(F,xi_r0);\n\np_liq=refpropm('P','T',T6+273.15,'Q',0,'ammonia','water',[xi_r 1-xi_r])/100;\ncatch\nxi_r=1\np_liq=refpropm('P','T',T6+273.15,'Q',0,'ammonia','water',[xi_r 1-xi_r])/100;\nend"("T7"=w555, "T6a"=w554, "T13"=w553, "T14"=w552, "xi_a"=w543, "p7"=w551, "p14"=w550, "T6"=w547) -> ("xi_r"=w549:dbl, "p_liq"=w546:dbl)  [unwired: 1 in, 1 out]
          }
        }
        "xi_r" <- w322
        "p_liq" <- w312
        n202 = Index Array(array=w272, index=13) -> (element=w274:dbl)
        n203 = Index Array(array=w212, index=22) -> (element=w247:dbl)
        n204 = call "Filter9"("Signal"=w312) -> ("Filtered Signal"=w310:dynamicdata)  [unwired: 9 in, 1 out]
        "p_liq_mittel" <- w310
        n205 = call "Pumpensteuerung_PID.vi"("reinitialize? (F)"="reinitialize Pumpe", "PID Regelung Pumpe"="PID Regelung Pumpe", "FI13 SW in l/min"="FI13 SW in l/min", "Prozessvariable"=w274, "Pumpensteuerung"="Pumpensteuerung") -> ("upper limit"=w317:dbl)  [unwired: 4 in, 2 out]
        n206 = call "Senkenregler_PID.vi"("Regelventil 36"="Regelventil 36", "Solltemp."="TI35 SW", "Regelventil 34"="Regelventil 34", "Regler Senke"="Regler Senke", "reinitialize?"="reinitialize Senke", "Numeric"=w247) -> ("upper limit 2"=w326:dbl, "upper limit"=w324:dbl)  [unwired: 6 in, 2 out]
        n207 = Greater?(x=w310, y=15.0) -> (0:w309:dynamicdata)
        n208 = case shown="True" w309 {
          tunnel: [w535 15.0 ("y")] -> w308
          tunnel: w309 -> [w535 _]
          frame False {
          }
          frame True {
          }
        }
        n209 = call "Filter7"("Signal"=w317) -> ("Filtered Signal"=w316:dynamicdata)  [unwired: 9 in, 1 out]
        "Mittelwert" <- w316
        n210 = Add(x="zusätzlicher Druck", y=w308) -> (x+y=w307:dynamicdata)
        n211 = case shown="True" "Mittelwert Pumpe" {
          tunnel: w317 -> [w539 _]
          tunnel: [w539 w540] -> w318
          tunnel: w316 -> [_ w540]
          frame False {
          }
          frame True {
          }
        }
        n212 = Greater Than 0?(x="RV 33") -> (x > 0?=w354:bool)
        n213 = Less Than 0?(x="RV 33") -> (x < 0?=w353:bool)
        n214 = Select(t=w487, s=w353, f=w488) -> (s? t:f=w485:i32)
        n215 = Select(t=w487, s=w354, f=w488) -> (s? t:f=w486:i32)
        n216 = call "Hochdruckregler_PID.vi"("Regler Hochdruck"="Regler Hochdruck", "Steuereingang"=w307, "Solldruck"="PI05 SW", "PI05"=w272, "Exp.V"="Exp.V", "reinitialize? (F) in"="reinitialize HD") -> ("upper limit out"=w249:dbl)  [unwired: 7 in, 2 out]
        n217 = call "Filter8"("Signal"=w249) -> ("Filtered Signal"=w313:dynamicdata)  [unwired: 9 in, 1 out]
        "Mittelwert 2" <- w313
        n218 = case shown="True" "Mittelwert HD" {
          tunnel: w249 -> [w537 _]
          tunnel: [w537 w538] -> w314
          tunnel: w313 -> [_ w538]
          frame False {
          }
          frame True {
          }
        }
        n219 = call "Stellungen_Namen2.vi"("Kühlventil"=w326, "Pumpensteuerung"=w318, "Regelventil 39"="Regelventil 39", "Exp.V"=w314, "Regelventil 14"=w324, "Meter"=w236, "zu"="RV 30 zu", "auf"="RV 30 auf", "Regelventil 35"="Regelventil 35") -> ("Dynamic Data"=w385:dynamicdata)  [unwired: 2 in]
        n220 = Build Array("PI05 SW", "TI35 SW", "FI13 SW in l/min") -> (w243:dbl[])
        n221 = Merge Signals(w385, w486, w485) -> (w250:dynamicdata)
        n222 = Insert Into Array(array=w211, new element=w243) -> (w213:dbl[])  [unwired: 1 in]
        n223 = call-poly <vilib>:"DAQmx Write.vi"("task/channels in"=w252, "auto start"=w253, "data"=w250, "error in"=w251) -> ()  [unwired: 9 in, 3 out]
        n224 = Index Array(array=w212, index=18) -> (element=w377:dbl)
        n225 = Index Array(array=w272, index #1=1, index #2=0, index #3=7, index #4=6) -> (element #1=w374:dbl, element #2=w373:dbl, element #3=w372:dbl, element #4=w371:dbl)
        n226 = Index Array(array=w213, index=0) -> (element=w305:dbl)
        n227 = Not Equal To 0?(x=w305) -> (x != 0?=w222:bool)
        n228 = Divide(x=w374, y=w373) -> (x/y=w493:dbl)
        "Druckverhältnis" <- w493
        n229 = Subtract(x=w372, y=w371) -> (x-y=w503:dbl)
        n230 = Greater?(x=w503, y=1.0) -> (0:w379:bool)
        "Fl.Pumpe an" <- w379
        n231 = feedback #3() -> (w220:dbl)  [unwired: 1 in]
        n232 = Select(t=w220, s=w222, f=w214) -> (s? t:f=w221:dbl)
        n233 = feedback-in #3(w221) -> ()
        n234 = Less?(x=w377, y=60) -> (x < y?=w439:bool)
        "Temperatur Öl" <- w439
        n235 = Greater?(x=w493, y=1.5) -> (0:w491:bool)
        n236 = feedback #4(w214) -> (w215:dbl)
        n237 = Select(t=w214, s="Reset", f=w215) -> (s? t:f=w216:dbl)
        n238 = feedback-in #4(w216) -> ()
        n239 = Subtract(x=w214, y=w221) -> (x-y=w219:dbl)
        n240 = Subtract(x=w214, y=w216) -> (x-y=w218:dbl)
        n241 = expression code="x-3600"(w219) -> (w496:dbl)
        n242 = Build Array(w439, w491) -> (→"Warnungen":bool[])
        n243 = expression code="x-3600"(w218) -> (w498:dbl)
        n244 = Greater?(x=w219, y=720.0) -> (0:w380:bool)
        "Magnetventil" <- w380
        n245 = Build Array(w222, w380, w379) -> (→"Status Komponenten":bool[])
        n246 = call "Verdichternamen.vi"("Array"=w213) -> ("Dynamic Data"=w494:dynamicdata)  [unwired: 10 in]
        n247 = Seconds To Date/Time(time stamp (now)=w496) -> (date time rec=w440:T15)  [unwired: 1 in]
        n248 = Seconds To Date/Time(time stamp (now)=w498) -> (date time rec=w507:T15)  [unwired: 1 in]
        n249 = Unbundle By Name(w507) -> ("second"=w506:i32, "minute"=w505:i32, "hour"=w499:i32)
        n250 = Unbundle By Name(w440) -> ("second"=w509:i32, "minute"=w508:i32, "hour"=w497:i32)
        n251 = Bundle("second"=w509, "minute"=w508, "hour"=w497) -> (→"Verdichteraktivität":cluster{"second":i32, "minute":i32, "hour":i32})  [unwired: 1 in]
        n252 = Bundle("second"=w506, "minute"=w505, "hour"=w499) -> (→"Betriebszeit":cluster{"second":i32, "minute":i32, "hour":i32})  [unwired: 1 in]
        n253 = Merge Signals(w267, w266, w385, w494) -> (w404:dynamicdata)
        n254 = flat-sequence {
          tunnel: [w598] -> w517
          tunnel: [w597] -> w516
          tunnel: w421 -> [w596]
          tunnel: w420 -> [w595]
          tunnel: [w593] -> w417
          tunnel: "Identität!" -> [w592]
          tunnel: "Dateiname!" -> [w591]
          tunnel: "Speichern" -> [w590]
          tunnel: "tag" -> [w589]
          tunnel: w517 -> [w696]
          tunnel: w516 -> [w695]
          tunnel: [w691] -> w424
          tunnel: [w693] -> w423
          tunnel: w422 -> [w692]
          frame #0 {
            n255 = Index Array(array=w595) -> (element=w594:timestamp)  [unwired: 1 in]
            n256 = event shown="[1] \"Speichern\": Value Change" {
              selector: _ -> [_ _ _]
              dyn-events: _ -> [_ _ _]
              timeout: 5 -> [_ _ _]
              tunnel: [_ w608 _] -> w598
              tunnel: w596 -> [_ w603 _]
              tunnel: ["" w607 ""] -> w597
              tunnel: w594 -> [_ w606 w677]
              tunnel: [_ _ w675] -> w593
              tunnel: w592 -> [_ w605 _]
              tunnel: w591 -> [_ w604 _]
              tunnel: w590 -> [_ w602 _]
              tunnel: w589 -> [_ w601 _]
              event Timeout {
                n257 = event-data() -> ()  [unwired: 1 in, 1 out]
              }
              event "Speichern": Value Change {
                n258 = event-data() -> ()  [unwired: 1 in, 1 out]
                n259 = case shown="False" w602 {
                  tunnel: [w640 _] -> w608
                  tunnel: [w635 _] -> w607
                  tunnel: w606 -> [w627 _]
                  tunnel: w605 -> [w611 _]
                  tunnel: w604 -> [w623 _]
                  tunnel: w603 -> [w622 _]
                  tunnel: w601 -> [w610 _]
                  frame False {
                    w614 = "\r"
                    n260 = property on="Dateiname!" class="Str"("DisabledEnum"=T4."Disabled and Grayed Out" ("Disabled")) -> ()  [unwired: 2 in, 2 out]
                    n261 = for {
                      N: 1 -> [_]
                      tunnel: ["Zeit"] -> w620 mode=indexing
                      tunnel: ["Kommentar"] -> w616 mode=indexing
                    }
                    n262 = Format Date/Time String(time format string (%c)="%d-%m-%Y_%H.%M ", seconds (now)=w627) -> (date/time string=w628:string)  [unwired: 1 in]
                    n263 = Concatenate Strings(w611, "\\", w628, w623, ".lvm" ("string")) -> (w630:string)
                    n264 = Insert Into Array(array=w622, index (row)=0, new element=w620) -> (w618:string[][])  [unwired: 1 in]
                    n265 = Build Path(base path=path "\\\\pcift88\\Studenten/HT-Waermepumpe/Messdaten" ("file path (dialog if empty)"), name or relative path=w630) -> (appended path=w625:path)
                    n266 = Concatenate Strings(w611, "\t", "tag: " ("string"), w610) -> (w609:string)
                    n267 = Insert Into Array(array=w618, new element=w616) -> (w617:string[][])  [unwired: 2 in]
                    n268 = Open/Create/Replace File(file path (use dialog)=w625, operation (0:open)=T11."replace or create with confirmation") -> (refnum out=→"refnum out":refnum<file>, error out=w640:errorcluster)  [unwired: 4 in, 1 out]
                    n269 = Transpose 2D Array(2D array=w617) -> (transposed array=w638:string[][])
                    n270 = Format Date/Time String(seconds (now)=w627) -> (date/time string=w637:string)  [unwired: 2 in]
                    n271 = Strip Path(path=w625) -> (name=w624:string)  [unwired: 1 out]
                    n272 = Array To Spreadsheet String(array=w638, 3:"%s" ("format string")) -> (spreadsheet string=w636:string)  [unwired: 1 in]
                    n273 = Concatenate Strings(w609, w614, w614, w624, w614, w614, w637, w614, w614, w636, w614, w614) -> (w635:string)
                  }
                  frame True {
                    n274 = local read "refnum out"() -> (w644:refnum<file>)
                    n275 = property on="Dateiname!" class="Str"("DisabledEnum"=T4."Enabled" ("Disabled")) -> ()  [unwired: 2 in, 2 out]
                    n276 = Close File(refnum=w644) -> ()  [unwired: 1 in, 2 out]
                  }
                }
              }
              event "Comment": Value Change {
                # "Umlaute + ß ersetzen, quick&dirty 4.1.2016"
                n277 = event-data() -> ()  [unwired: 1 in, 1 out]
                n278 = flat-sequence {
                  tunnel: ["Kommentar"] -> w645
                  tunnel: w677 -> [w681]
                  frame #0 {
                    w683 = "\r"
                    n279 = local read "Historie"() -> (w685:string)
                    n280 = Get Date/Time String(seconds (now)=w681, want seconds? (F)=TRUE) -> (time string=w684:string)  [unwired: 1 in, 1 out]
                    n281 = Concatenate Strings(w685, w684, " -> ", "Kommentar", w683, w683) -> (→"Historie":string)
                  }
                  frame #1 {
                    n282 = local write "Kommentar"("") -> ()
                  }
                }
                n283 = Search and Replace String(replace all?=TRUE, input string=w645, search string="ä", replace string="ae") -> (result string=w667:string)  [unwired: 4 in, 3 out]
                n284 = Search and Replace String(replace all?=TRUE, input string=w667, search string="ü", replace string="ue") -> (result string=w666:string)  [unwired: 4 in, 3 out]
                n285 = Search and Replace String(replace all?=TRUE, input string=w666, search string="ö", replace string="oe") -> (result string=w665:string)  [unwired: 4 in, 3 out]
                n286 = Search and Replace String(replace all?=TRUE, input string=w665, search string="ß", replace string="ss") -> (result string=w646:string)  [unwired: 4 in, 3 out]
                n287 = Search and Replace String(replace all?=TRUE, input string=w646, search string="Ä", replace string="Ae") -> (result string=w655:string)  [unwired: 4 in, 3 out]
                n288 = Search and Replace String(replace all?=TRUE, input string=w655, search string="Ü", replace string="Ue") -> (result string=w654:string)  [unwired: 4 in, 3 out]
                n289 = Search and Replace String(replace all?=TRUE, input string=w654, search string="Ö", replace string="Oe") -> (result string=w647:string)  [unwired: 4 in, 3 out]
                n290 = for {
                  N: 1 -> [_]
                  tunnel: [w678] -> w675 mode=indexing
                  tunnel: w647 -> [w678]
                }
              }
            }
          }
          frame #1 {
            n291 = local read "refnum out"() -> (w688:refnum<file>)
            n292 = Concatenate Strings(w695, w692) -> (w694:string)
            n293 = Not A Number/Path/Refnum?(number/path/refnum=w688) -> (NaN/Path/Refnum?=w689:bool)
            n294 = Set File Position(refnum=w688, from (0:start)=enum16{"start", "end", "current"}."end", error in=w696) -> (refnum out=w697:refnum<file>, error out=w698:errorcluster)  [unwired: 1 in]
            n295 = Not(x=w689) -> (.not. x?=→"Speichert!":bool)
            n296 = Write to Text File(file (use dialog)=w697, text=w694, error in=w698) -> (refnum out=w691:refnum<file>, error out=w693:errorcluster)  [unwired: 1 in, 1 out]
          }
        }
        n297 = Empty String/Path?(string/path="Identität!") -> (empty?=w415:bool)
        n298 = Empty String/Path?(string/path="Dateiname!") -> (empty?=w414:bool)
        n299 = local read "Keithley Temperature Graph"() -> (w207:waveform(dbl)[])
        n300 = Or(x=w415, y=w414) -> (x .or. y?=w411:bool)
        n301 = call "Protokollordnung"("Signals"=w404) -> ("Signal Out"=w429:dynamicdata)  [unwired: 9 in, 1 out]
        n302 = Boolean To (0,1)(Boolean=w411) -> (0, 1=w412:i16)
        n303 = expression code="x*2"(w412) -> (w413:i16)
        n304 = call "Convert from Dynamic Data"("Dynamic Data Type"=w429) -> ("Array of Waveform"=w209:waveform(dbl)[])  [unwired: 3 in]
        n305 = property on="Speichern" class="Bool (strict)"("DisabledEnum"=w413) -> ()  [unwired: 2 in, 2 out]
        n306 = Insert Into Array(array=w209, new element=w207) -> (w208:waveform(dbl)[])  [unwired: 1 in]
        n307 = Array Size(array=w208) -> (size(s)=w407:i32)
        n308 = Concatenate Strings("%" ("string"), "." ("string"), ";%g" ("string")) -> (w431:string)
        n309 = Initialize Array(w431, w407) -> (w430:string[])
        n310 = for {
          tunnel: w208 -> [w702] mode=indexing
          tunnel: [w709] -> w427 mode=indexing
          tunnel: w430 -> [w707] mode=indexing
          tunnel: [w701] -> w421 mode=indexing
          tunnel: [w703] -> w420 mode=indexing
          tunnel: [w704] -> w426 mode=indexing
          n311 = Unbundle By Name(w702) -> ("Y"=w708:dbl[], "t0"=w700:timestamp)
          n312 = Get Waveform Attribute(5:w700, 6:"NI_ExpTimeStamp", 7:w702) -> (1:w703:timestamp)  [unwired: 1 in, 3 out]
          n313 = for {
            tunnel: w708 -> [w716] mode=indexing
            tunnel: [w715] -> w709 mode=indexing
            tunnel: w707 -> [w714]
            tunnel: w702 -> [w713]
            tunnel: [w712] -> w701 mode=indexing
            n314 = Format Into String(format string=w714, w716) -> (resulting string=w715:string)  [unwired: 2 in, 1 out]
            n315 = Get Waveform Attribute(5:"", 6:"NI_ChannelName", 7:w713) -> (1:w712:string)  [unwired: 1 in, 3 out]
          }
          n316 = Format Date/Time String(time format string (%c)="%H.%M.%S", seconds (now)=w703) -> (date/time string=w704:string)  [unwired: 1 in]
        }
        n317 = Insert Into Array(array=w427, index (row)=0, new element=w426) -> (w418:string[][])  [unwired: 1 in]
        n318 = Increment(x=w407) -> (x+1=w408:i32)
        n319 = Insert Into Array(array=w418, index (row)=w408, new element=w417) -> (w419:string[][])  [unwired: 1 in]
        n320 = Transpose 2D Array(2D array=w419) -> (transposed array=w416:string[][])
        n321 = Array To Spreadsheet String(array=w416, 3:"%s" ("format string")) -> (spreadsheet string=w422:string)  [unwired: 1 in]
        n322 = local write "stop"("Programm stoppen!") -> ()
      }
      frame #2 {
        n323 = Tick Count (ms)() -> (millisecond timer value=w834:u32)
        n324 = Subtract(x=w834, y=w833) -> (x-y=w832:u32)
        n325 = Divide(x=w832, y=1000.0) -> (x/y=→"Schleifendauer":dbl)
      }
    }
  }
  n326 = call <vilib>:"DAQmx Clear Task.vi"("task in"=w23, "error in"=w21) -> ()  [unwired: 13 in, 1 out]
  n327 = call <vilib>:"DAQmx Clear Task.vi"("task in"=w22, "error in"=w20) -> ()  [unwired: 13 in, 1 out]
  n328 = Merge Errors(w16) -> (w15:errorcluster)
  n329 = Close File(refnum=w47, error in=w15) -> (error out=w50:errorcluster)  [unwired: 1 out]
  n330 = call <vilib>:"General Error Handler.vi"("error in (no error)"=w50, "[exception action] (none:0)"=1 ("[exception code]"), "[exception code]"=1) -> ()  [unwired: 8 in, 5 out]
